vi "Stilts Calculations.vi"(2 "Pitch":dbl, 3 "Roll":dbl, 4 "Climb":dbl) -> (0 "Right":dbl, 1 "Left":dbl)   [LabVIEW 2018]
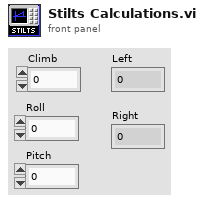
[diagram p1: front panel]
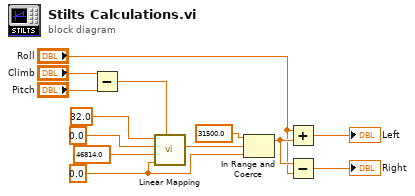
[diagram p0: block diagram]
diagram:
  w12 = 0.0 ("Min B")
  n1 = Subtract(x="Climb", y="Pitch") -> (x-y=w7:dbl)
  n2 = call "Linear Mapping.vi"("X"=w7, "Min B"=w12, "Max B"=46814.0, "Min A"=0.0, "Max A"=32.0) -> ("Y"=w10:dbl)  [unwired: 6 in]
  n3 = In Range and Coerce(upper limit=31500.0, x=w10, lower limit=w12) -> (coerced(x)=w9:dbl)  [unwired: 1 out]
  n4 = Add(x="Roll", y=w9) -> (x+y=→"Left":dbl)
  n5 = Subtract(x=w9, y="Roll") -> (x-y=→"Right":dbl)
